vi "Measurement Logic.vi"() -> ()   [LabVIEW 2021, in "Z Power Module.lvlib"]
uses:
  Z Power Module.lvlib
  Measurement Configuration.ctl
  Measurement Results.ctl
  <vilib>/Plug-In SDKs/Measurements/Measure Call Context/Measure Call Context.lvclass
panel:
  out "measure call context out":refnum<class "Measure Call Context.lvclass">
  in  "measure call context in":refnum<class "Measure Call Context.lvclass">
  out "measurement results":T1
  in  "measurement configuration":T2={"Calculate Analysis?"=TRUE, "Current Setpoint"=1.2, "Voltage Setpoint"=0.0, "Physical Channel"="Lorem ipsum dolor sit"}
  out "error out":errorcluster
  in  "error in":errorcluster
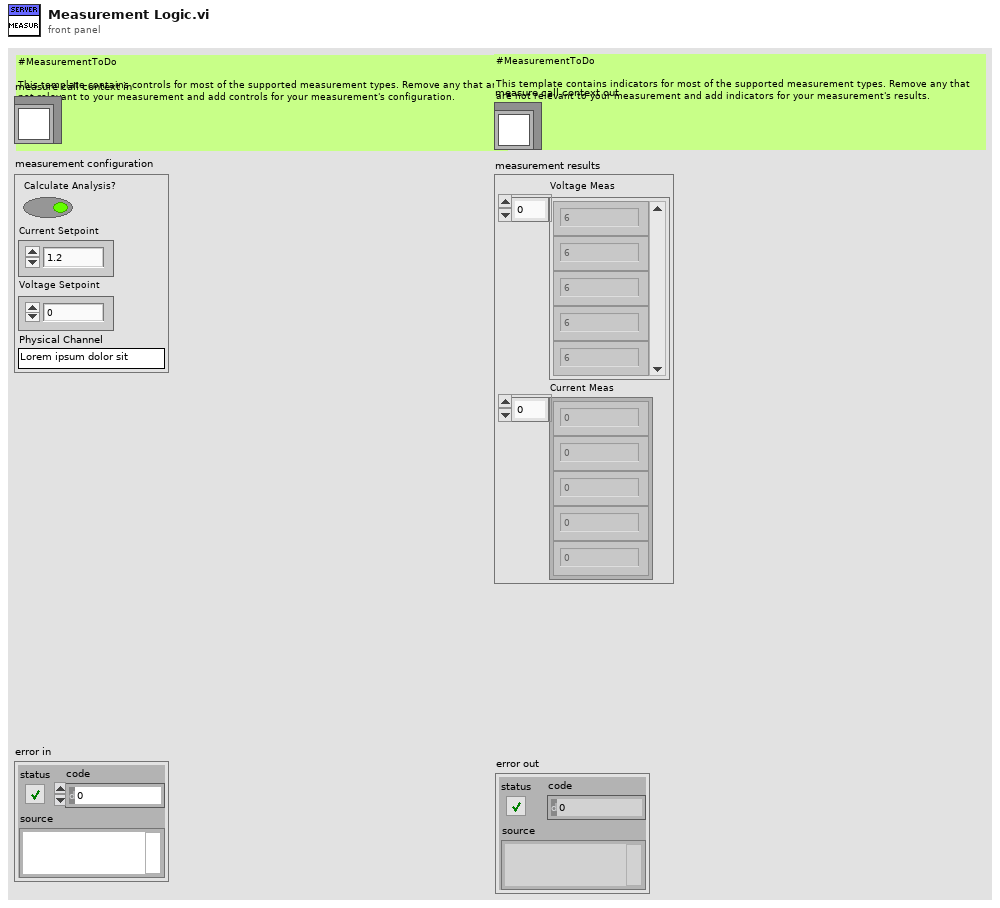
[diagram p1: front panel]
types:
  T1 = typedef "Z Power Module.lvlib/Measurement Results.ctl" = cluster{"Voltage Meas":dbl[], "Current Meas":dbl[]}
  T2 = typedef "Z Power Module.lvlib/Measurement Configuration.ctl" = cluster{"Calculate Analysis?":bool, "Current Setpoint":dbl, "Voltage Setpoint":dbl, "Physical Channel":string}
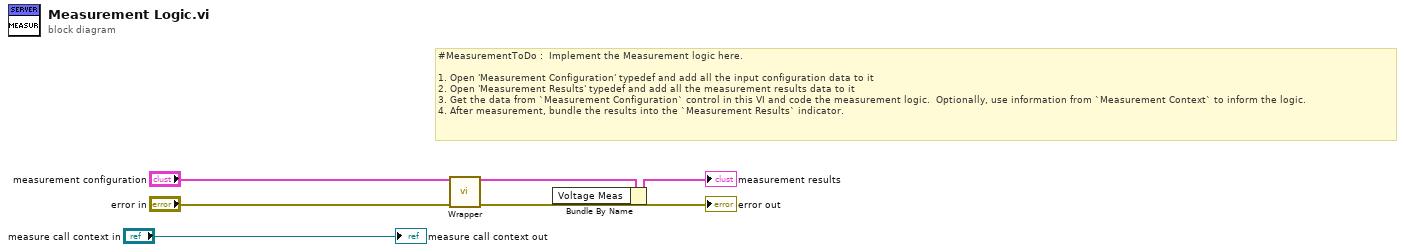
[diagram p0: block diagram]
diagram:
  # "#MeasurementToDo :  Implement the Measurement logic here.\n\n1. Open 'Measurement Configuration' typedef and add all the input configuration data to it\n2. Open 'Measurement Results' typedef and add all the measurement results data to it\n3. Get the data from `Measurement Configuration` control in this VI and code the measurement logic.  Optionally, use information from `Measurement Context` to inform the logic.\n4. After measurement, bundle the results into the `Measurement Results` indicator."
  n1 = call "Wrapper.vi"("measurement configuration"="measurement configuration", "error in"="error in") -> ("measurement results"=w5:T1, "error out"=→"error out":errorcluster)  [unwired: 12 in]
  n2 = Bundle By Name(cluster=w5) -> (→"measurement results":T1)  [unwired: 1 in]
  "measure call context out" <- "measure call context in"
